vi "Power Accuracy Display Key Array.vi"(4 "Conversion":enum16{"Cluster - HTML", "HTML - Cluster"}(ring), 6 "Display Key Array In":T2, 7 "Display Cluster In":T1={"Power"={"Min"=-160, "Max"=-60}, "Tolerance"={"Min"=0.0, "Max"=0.0}}) -> (1 "Display Cluster Out":T1={"Power"={"Min"=-160, "Max"=-60}, "Tolerance"={"Min"=0.0, "Max"=0.0}}, 2 "Display HTML Out":string)   [LabVIEW 2011]
uses:
  ITK EXT/utils/keyedarr.llb/Keyed Array.ctl
  TypeDefs/Power Accuracy Display Parameters.ctl
  ITK EXT/utils/strutil.llb/Case Matching.ctl
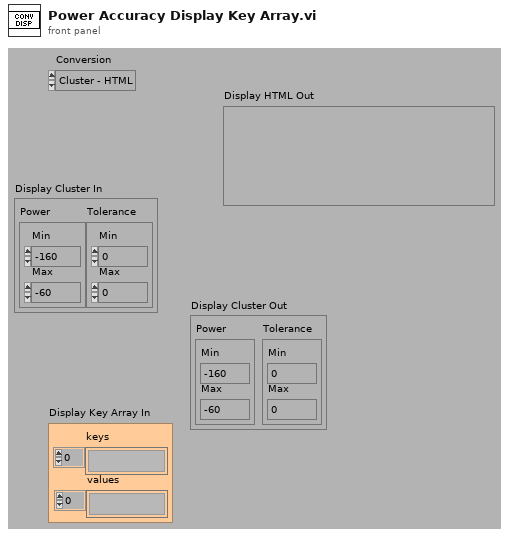
[diagram p1: front panel]
types:
  T1 = typedef "Power Accuracy Display Parameters.ctl" = cluster{"Power":cluster{"Min":i32, "Max":i32}, "Tolerance":cluster{"Min":dbl, "Max":dbl}}
  T2 = typedef "Keyed Array.ctl" = cluster{"keys":string[], "values":string[]}
  T3 = typedef "Case Matching.ctl" = enum16{"a != A", "a == A", "system"}
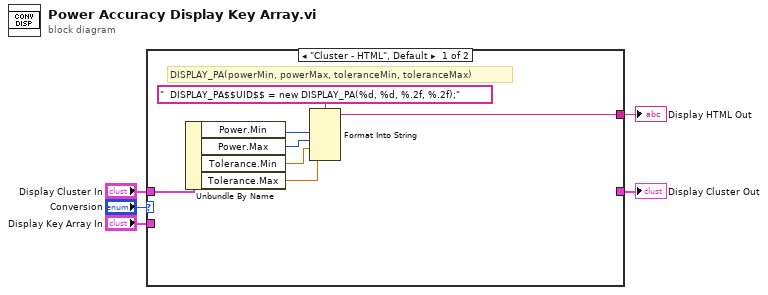
[diagram p0: block diagram]
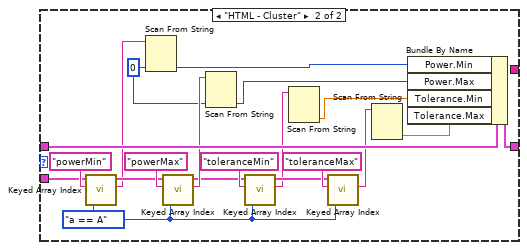
[diagram p2: hidden frame]
diagram:
  n1 = case shown="\"Cluster - HTML\", Default" "Conversion" {
    tunnel: "Display Key Array In" -> [_ w14]
    tunnel: "Display Cluster In" -> [w12 w32]
    tunnel: [w7 _] -> w3
    tunnel: [_ w31] -> w2
    frame "Cluster - HTML", Default {
      # "DISPLAY_PA(powerMin, powerMax, toleranceMin, toleranceMax)"
      n2 = Unbundle By Name(w12) -> ("Power.Min"=w10:i32, "Power.Max"=w9:i32, "Tolerance.Min"=w8:dbl, "Tolerance.Max"=w6:dbl)
      n3 = Format Into String(format string="  DISPLAY_PA$$UID$$ = new DISPLAY_PA(%d, %d, %.2f, %.2f);", w10, w9, w8, w6) -> (resulting string=w7:string)  [unwired: 2 in, 1 out]
    }
    frame "HTML - Cluster" {
      w22 = 0 ("Measure.Ref Units")
      w13 = Case_Matching."a == A" ("case matching (sensitive)")
      n4 = call "Keyed Array Index.vi"("case matching (sensitive)"=w13, "key"="powerMin", "array in"=w14) -> ("value"=w24:string, "duplicate array"=w28:T2)  [unwired: 1 in, 2 out]
      n5 = Scan From String(input string=w24, default 1=w22) -> (output 1=w25:i32)  [unwired: 3 in, 3 out]
      n6 = call "Keyed Array Index.vi"("case matching (sensitive)"=w13, "key"="powerMax", "array in"=w28) -> ("value"=w23:string, "duplicate array"=w20:T2)  [unwired: 1 in, 2 out]
      n7 = Scan From String(input string=w23, default 1=w22) -> (output 1=w21:i32)  [unwired: 3 in, 3 out]
      n8 = call "Keyed Array Index.vi"("case matching (sensitive)"=w13, "key"="toleranceMin", "array in"=w20) -> ("value"=w18:string, "duplicate array"=w19:T2)  [unwired: 1 in, 2 out]
      n9 = Scan From String(input string=w18) -> (output 1=w17:dbl)  [unwired: 3 in, 4 out]
      n10 = call "Keyed Array Index.vi"("case matching (sensitive)"=w13, "key"="toleranceMax", "array in"=w19) -> ("value"=w16:string)  [unwired: 1 in, 3 out]
      n11 = Scan From String(input string=w16) -> (output 1=w15:dbl)  [unwired: 3 in, 4 out]
      n12 = Bundle By Name(cluster=w32, "Power.Min"=w25, "Power.Max"=w21, "Tolerance.Min"=w17, "Tolerance.Max"=w15) -> (w31:T1)
    }
  }
  "Display HTML Out" <- w3
  "Display Cluster Out" <- w2
